vi "LWXPS_GatheringUserDatasGet.vi"(1 "XPS Reference IN":refnum<k24>, 6 "LabVIEW error IN":errorcluster) -> (8 "XPS Reference OUT":refnum<k24>, 9 "LabVIEW error OUT":errorcluster, 10 "Returned error code":i32, 11 "XPS Error String":string, 12 "User Data 1":dbl, 13 "User Data 16":dbl, 14 "User Data 2":dbl, 15 "User Data 15":dbl, 16 "User Data 3":dbl, 17 "User Data 14":dbl, 18 "User Data 4":dbl, 19 "User Data 13":dbl, 20 "User Data 5":dbl, 21 "User Data 6":dbl, 22 "User Data 7":dbl, 23 "User Data 8":dbl, 24 "User Data 9":dbl, 25 "User Data 10":dbl, 26 "User Data 11":dbl, 27 "User Data 12":dbl)   [LabVIEW 2014]
uses:
  D:/XPSQ8_LabView_Library/Development/Source/Dll/Newport.XPS.CommandInterface.dll
  Dll/Newport.XPS.CommandInterface.dll
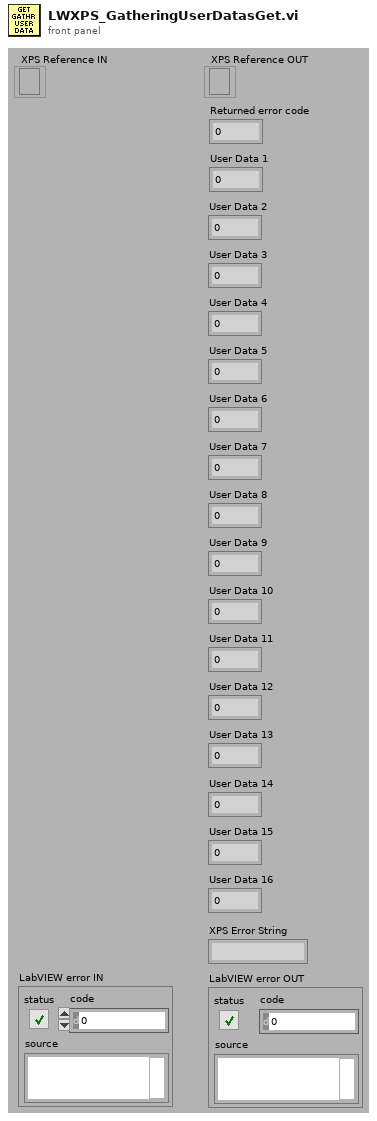
[diagram p1: front panel]
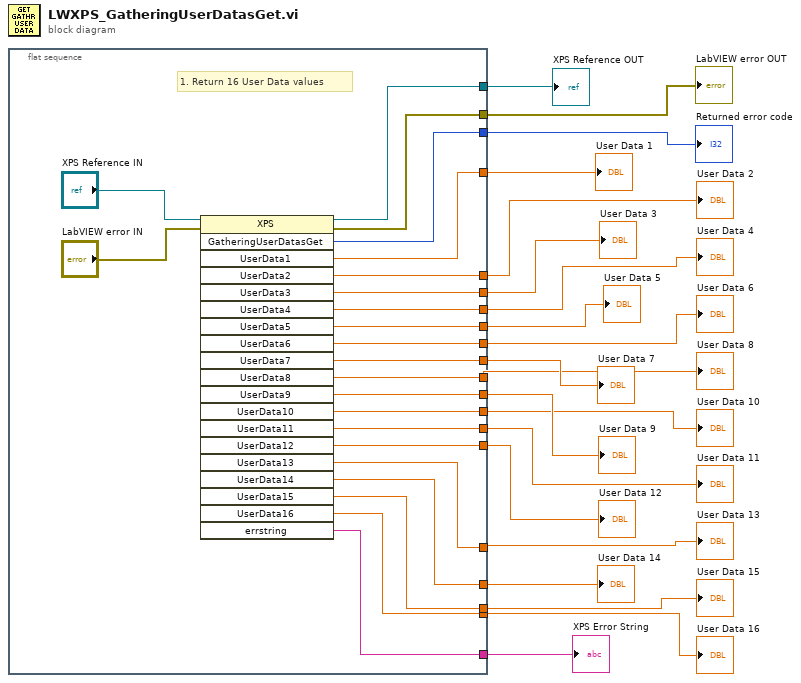
[diagram p0: block diagram]
diagram:
  n1 = flat-sequence {
    tunnel: [w38] -> w20
    tunnel: [w42] -> w19
    tunnel: [w41] -> w2
    tunnel: [w37] -> w18
    tunnel: [w36] -> w6
    tunnel: [w35] -> w4
    tunnel: [w34] -> w7
    tunnel: [w33] -> w8
    tunnel: [w32] -> w9
    tunnel: [w31] -> w15
    tunnel: [w30] -> w17
    tunnel: [w29] -> w16
    tunnel: [w28] -> w14
    tunnel: [w27] -> w1
    tunnel: [w26] -> w5
    tunnel: [w25] -> w13
    tunnel: [w24] -> w12
    tunnel: [w23] -> w11
    tunnel: [w21] -> w10
    tunnel: [w22] -> w3
    frame #0 {
      # "1. Return 16 User Data values"
      n2 = invoke class="XPS" method="GatheringUserDatasGet"(reference="XPS Reference IN", error in="LabVIEW error IN") -> (reference out=w38:refnum<k24>, error out=w42:errorcluster, "GatheringUserDatasGet"=w41:i32, "UserData1"=w36:dbl, "UserData2"=w35:dbl, "UserData3"=w34:dbl, "UserData4"=w33:dbl, "UserData5"=w32:dbl, "UserData6"=w31:dbl, "UserData7"=w30:dbl, "UserData8"=w29:dbl, "UserData9"=w28:dbl, "UserData10"=w27:dbl, "UserData11"=w26:dbl, "UserData12"=w25:dbl, "UserData13"=w24:dbl, "UserData14"=w23:dbl, "UserData15"=w22:dbl, "UserData16"=w21:dbl, "errstring"=w37:string)  [unwired: 18 in]
    }
  }
  "XPS Reference OUT" <- w20
  "LabVIEW error OUT" <- w19
  "Returned error code" <- w2
  "XPS Error String" <- w18
  "User Data 7" <- w17
  "User Data 8" <- w16
  "User Data 6" <- w15
  "User Data 9" <- w14
  "User Data 10" <- w1
  "User Data 11" <- w5
  "User Data 12" <- w13
  "User Data 13" <- w12
  "User Data 14" <- w11
  "User Data 15" <- w3
  "User Data 16" <- w10
  "User Data 5" <- w9
  "User Data 4" <- w8
  "User Data 3" <- w7
  "User Data 2" <- w4
  "User Data 1" <- w6
